vi "motor motion and reset.vi"(0 "VISA Refnum in":refnum<visa-resource-name>, 1 "Dup Controller # in":string, 5 "DELAY (ms) in":u32, 7 "Reset":bool, 9 "Move step size":i32, 11 "error in (no error)":errorcluster, 12 "Reset displacement":ext) -> (3 "DELAY (ms) out":u32, 4 "VISA Refnum out":refnum<visa-resource-name>, 6 "Dup Controller # out":string, 8 "ABSOLUTE DSPLACEMENT":i64, 10 "Response":string, 15 "error out":errorcluster)   [LabVIEW 2014]
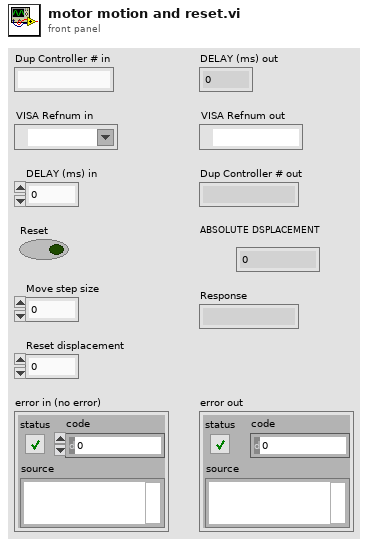
[diagram p1: front panel]
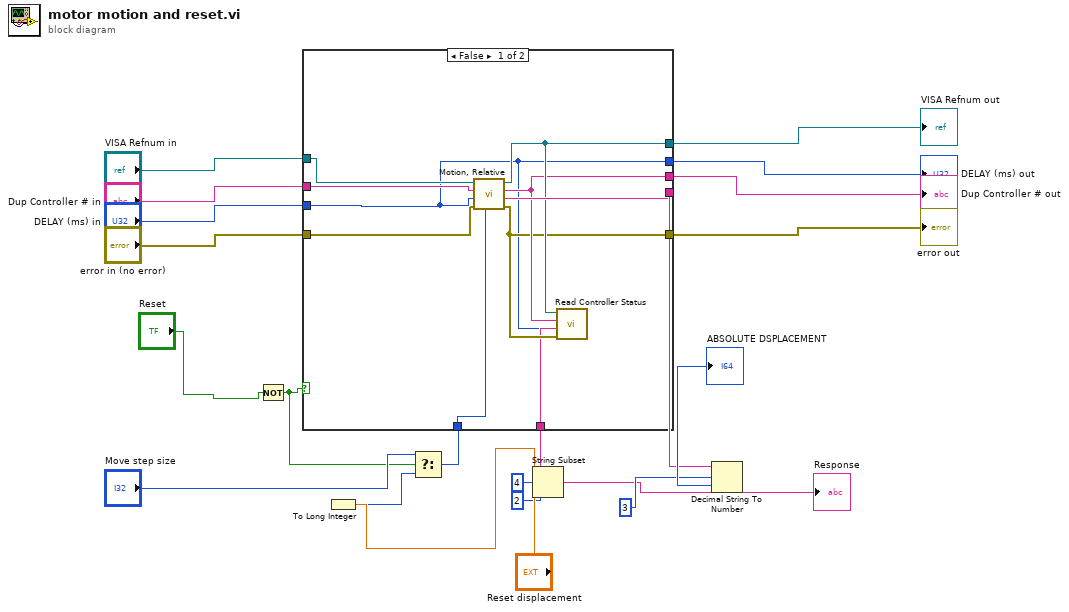
[diagram p0: block diagram]
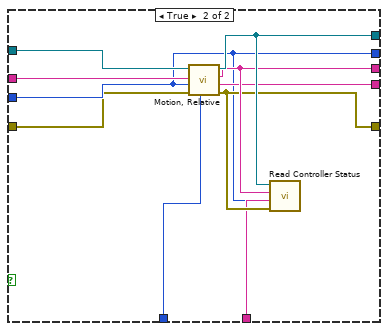
[diagram p2: hidden frame]
diagram:
  n1 = Not(x="Reset") -> (.not. x?=w16:bool)
  n2 = To Long Integer(number="Reset displacement") -> (32bit integer=w17:i32)
  n3 = Select(t="Move step size", s=w16, f=w17) -> (s? t:f=w20:i32)
  n4 = case shown="False" w16 {
    tunnel: "VISA Refnum in" -> [w26 w36]
    tunnel: "Dup Controller # in" -> [w25 w35]
    tunnel: "DELAY (ms) in" -> [w24 w34]
    tunnel: "error in (no error)" -> [w23 w33]
    tunnel: w20 -> [w22 w32]
    tunnel: [w30 w41] -> w13
    tunnel: [w29 w40] -> w14
    tunnel: [w24 w34] -> w12
    tunnel: [w28 w39] -> w15
    tunnel: [w31 w37] -> w9
    tunnel: [w27 w38] -> w5
    frame False {
      n5 = call <userlib>:"Motion, Relative.vi"("Value"=w22, "error in (no error)"=w23, "Delay (ms)"=w24, "Controller #"=w25, "VISA Handle"=w26) -> ("error out"=w28:errorcluster, "Response"=w31:string, "Dup Controller #"=w29:string, "Dup VISA Handle"=w30:refnum<visa-resource-name>)  [unwired: 1 in, 1 out]
      n6 = call <userlib>:"Read Controller Status.vi"("error in (no error)"=w28, "Delay (ms)"=w24, "Controller #"=w29, "VISA Handle"=w30) -> ("Response"=w27:string)  [unwired: 5 out]
    }
    frame True {
      n7 = call <userlib>:"Motion, Relative.vi"("Value"=w32, "error in (no error)"=w33, "Delay (ms)"=w34, "Controller #"=w35, "VISA Handle"=w36) -> ("error out"=w39:errorcluster, "Response"=w37:string, "Dup Controller #"=w40:string, "Dup VISA Handle"=w41:refnum<visa-resource-name>)  [unwired: 1 in, 1 out]
      n8 = call <userlib>:"Read Controller Status.vi"("error in (no error)"=w39, "Delay (ms)"=w34, "Controller #"=w40, "VISA Handle"=w41) -> ("Response"=w38:string)  [unwired: 5 out]
    }
  }
  "error out" <- w15
  "Dup Controller # out" <- w14
  "VISA Refnum out" <- w13
  "DELAY (ms) out" <- w12
  n9 = String Subset(string=w5, offset (0)=4, length (rest)=2 ("length (rest)")) -> (substring=→"Response":string)
  n10 = Decimal String To Number(string=w9, offset=3) -> (number=→"ABSOLUTE DSPLACEMENT":i32)  [unwired: 2 out]
